vi "Write formattedOutputData.vi"(10 "formattedOutputData":string, 11 "ILC in":refnum<class "ILC.lvclass">) -> (3 "ILC out":refnum<class "ILC.lvclass">)   [LabVIEW 2013]
uses:
  <userlib>/Common/ILC/ILC/ILC.lvclass
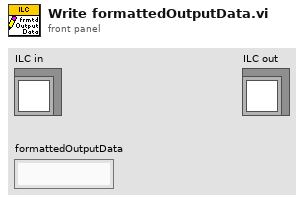
[diagram p1: front panel]
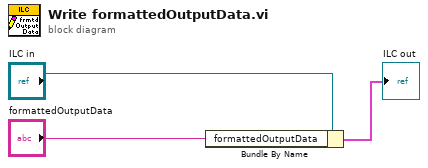
[diagram p0: block diagram]
diagram:
  n1 = Bundle By Name(cluster="ILC in", "formattedOutputData"="formattedOutputData") -> (→"ILC out":cluster{})
